vi "删除用户.vi"(6 "用户名-refnum-in":refnum<vi>, 8 "用户类别-refnum-in":refnum<vi>, 9 "管理人员1+密码":string[][](array[string]), 10 "操作人员0+密码":string[][](array[string]), 11 "密码文件路径":path=path "E:/LabVIEW Data/盾构/default") -> (2 "管理人员1+密码_out":string[][](array[string]), 3 "操作人员0+密码_out":string[][](array[string]))   [LabVIEW 2018]
panel:
  in  "用户名":u16(ring) caption="请在此选择用户名" items=["1", "2"]
  in  "用户类别":u8(ring) caption="请在此选择用户类别" items=["操作人员", "管理人员"]
  in  "请输入密码":string
  in  "返回":bool
  in  "删除":bool
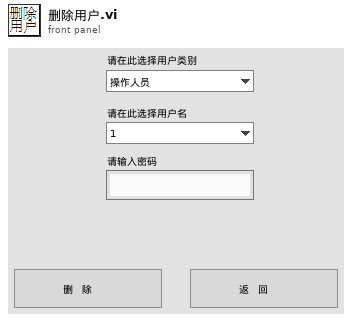
[diagram p1: front panel]
types:
  T1 = enum8{"Enabled", "Disabled", "Disabled and Grayed Out"}
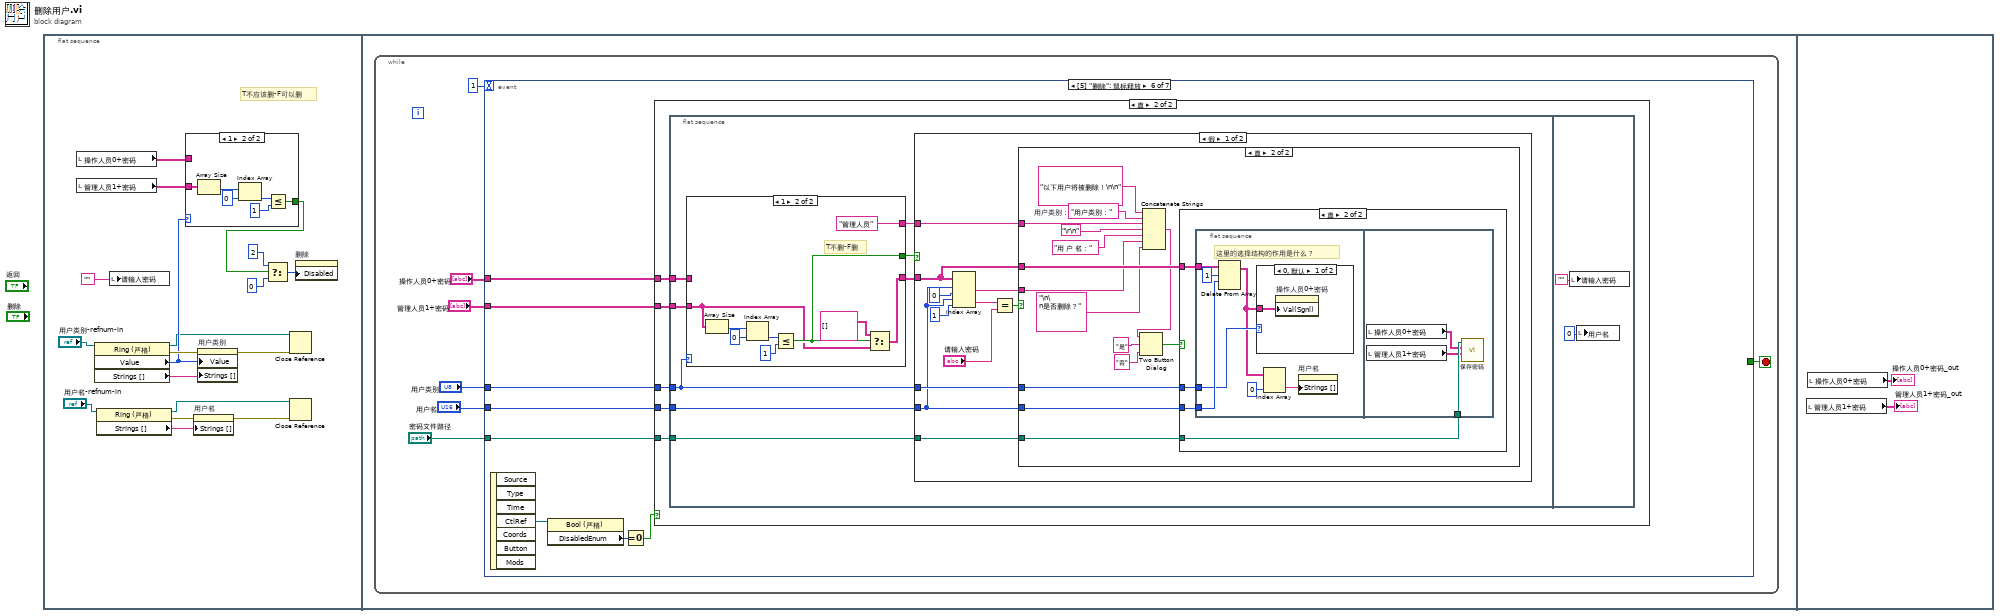
[diagram p0: block diagram]
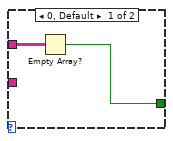
[diagram p2: hidden frame]
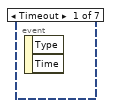
[diagram p3: hidden frame]
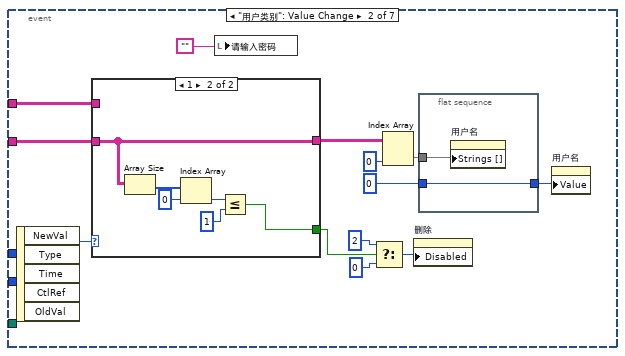
[diagram p4: hidden frame]
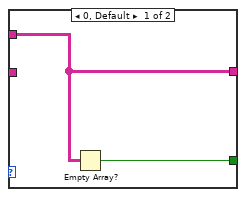
[diagram p5: hidden frame]
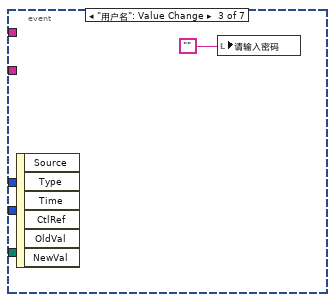
[diagram p6: hidden frame]
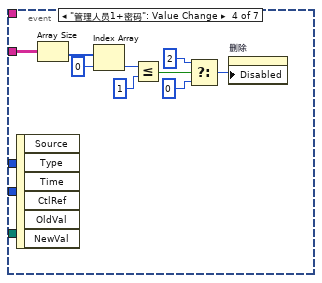
[diagram p7: hidden frame]
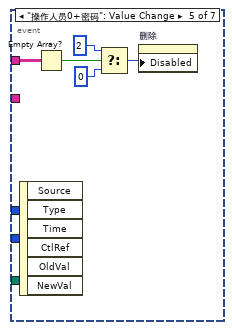
[diagram p8: hidden frame]
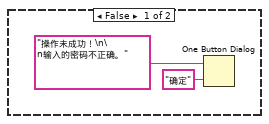
[diagram p10: hidden frame]
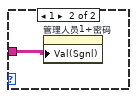
[diagram p12: hidden frame]
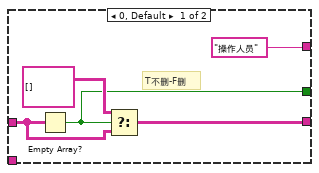
[diagram p14: hidden frame]
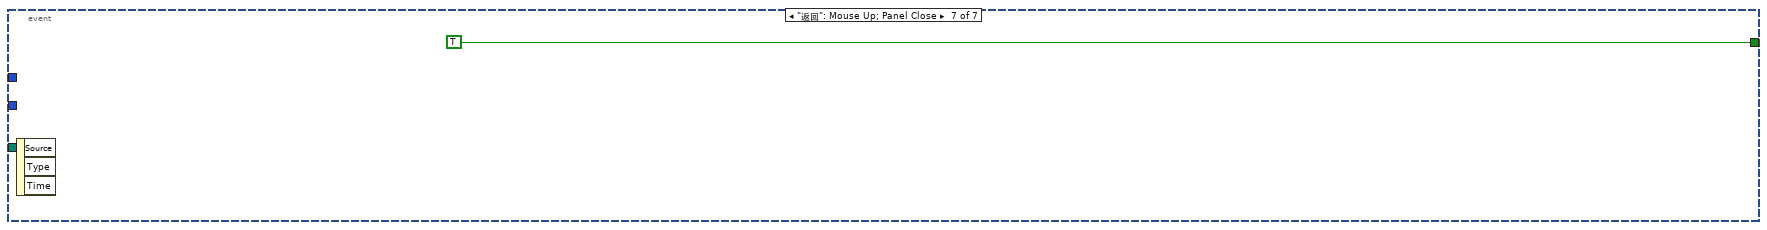
[diagram p15: hidden frame]
diagram:
  n1 = flat-sequence {
    frame #0 {
      # "T不应该删-F可以删"
      n2 = local read "操作人员0+密码"() -> (w10:string[][])
      n3 = local read "管理人员1+密码"() -> (w11:string[][])
      n4 = property class="Ring (严格)"(reference="用户类别-refnum-in") -> (reference out=w3:refnum<vi>, error out=w13:errorcluster, "Value"=w12:u8, "Strings []"=w17:string[])  [unwired: 1 in]
      n5 = property class="Ring (严格)"(reference="用户名-refnum-in") -> (reference out=w1:refnum<vi>, error out=w15:errorcluster, "Strings []"=w14:string[])  [unwired: 1 in]
      n6 = local write "请输入密码"("") -> ()
      n7 = case shown="1" w12 {
        tunnel: w10 -> [w20 _]
        tunnel: w11 -> [_ w21]
        tunnel: [w19 w22] -> w6
        frame 0, Default {
          n8 = Empty Array?(array=w20) -> (empty?=w19:bool)
        }
        frame 1 {
          n9 = Array Size(array=w21) -> (size(s)=w26:i32[])
          n10 = Index Array(array=w26, index=0 ("索引")) -> (element=w24:i32)
          n11 = Less Or Equal?(x=w24, y=1) -> (x <= y?=w22:bool)
        }
      }
      n12 = property on="用户名" class="Ring (严格)"(error in=w15, "Strings []"=w14) -> (error out=w2:errorcluster)  [unwired: 1 in, 1 out]
      n13 = property on="用户类别" class="Ring (严格)"(error in=w13, "Value"=w12, "Strings []"=w17) -> (error out=w4:errorcluster)  [unwired: 1 in, 1 out]
      n14 = Select(t=u8 2 ("禁用"), s=w6, f=u8 0 ("禁用")) -> (s? t:f=w7:u8)
      n15 = Close Reference(reference=w3, error in (no error)=w4) -> ()  [unwired: 1 out]
      n16 = Close Reference(reference=w1, error in (no error)=w2) -> ()  [unwired: 1 out]
      n17 = property on="删除" class="Bool (严格)"("Disabled"=w7) -> ()  [unwired: 2 in, 2 out]
    }
    frame #1 {
      n18 = while {
        stop <- w32 stop-if-true
        n19 = event shown="[5] \"删除\": 鼠标释放" {
          selector: _ -> [_ _ _ _ _ _ _]
          dyn-events: _ -> [_ _ _ _ _ _ _]
          timeout: 1 -> [_ _ _ _ _ _ _]
          tunnel: "操作人员0+密码" -> [_ w39 _ _ w71 w79 _]
          tunnel: "管理人员1+密码" -> [_ w38 _ w62 _ w78 _]
          tunnel: "用户类别" -> [_ _ _ _ _ w76 _]
          tunnel: "密码文件路径" -> [_ _ _ _ _ w75 _]
          tunnel: [_ _ _ _ _ _ TRUE] -> w32
          tunnel: "用户名" -> [_ _ _ _ _ w77 _]
          event Timeout {
            n20 = event-data() -> ()  [unwired: 1 in, 2 out]
          }
          event "用户类别": Value Change {
            n21 = event-data() -> ("NewVal"=w46:u8)  [unwired: 1 in, 4 out]
            n22 = case shown="1" w46 {
              tunnel: w39 -> [w50 _]
              tunnel: [w50 w52] -> w40
              tunnel: w38 -> [_ w52]
              tunnel: [w49 w51] -> w34
              frame 0, Default {
                n23 = Empty Array?(array=w50) -> (empty?=w49:bool)
              }
              frame 1 {
                n24 = Array Size(array=w52) -> (size(s)=w53:i32[])
                n25 = Index Array(array=w53, index=0 ("索引")) -> (element=w55:i32)
                n26 = Less Or Equal?(x=w55, y=1) -> (x <= y?=w51:bool)
              }
            }
            n27 = local write "请输入密码"("") -> ()
            n28 = Select(t=u8 2 ("禁用"), s=w34, f=u8 0 ("禁用")) -> (s? t:f=w35:u8)
            n29 = Index Array(array=w40, index (col)=0 ("禁用的索引 (col)")) -> (element=w45:string[])  [unwired: 1 in]
            n30 = property on="删除" class="Bool (严格)"("Disabled"=w35) -> ()  [unwired: 2 in, 2 out]
            n31 = flat-sequence {
              tunnel: w45 -> [w48]
              tunnel: [w47] -> w42
              tunnel: u16 0 ("禁用的索引 (col)") -> [w47]
              frame #0 {
                n32 = property on="用户名" class="Ring (严格)"("Strings []"=w48) -> ()  [unwired: 2 in, 2 out]
              }
            }
            n33 = property on="用户名" class="Ring (严格)"("Value"=w42) -> ()  [unwired: 2 in, 2 out]
          }
          event "用户名": Value Change {
            n34 = event-data() -> ()  [unwired: 1 in, 6 out]
            n35 = local write "请输入密码"("") -> ()
          }
          event "管理人员1+密码": Value Change {
            n36 = event-data() -> ()  [unwired: 1 in, 6 out]
            n37 = Array Size(array=w62) -> (size(s)=w63:i32[])
            n38 = Index Array(array=w63, index=0 ("索引")) -> (element=w65:i32)
            n39 = Less Or Equal?(x=w65, y=1) -> (x <= y?=w58:bool)
            n40 = Select(t=u8 2 ("禁用"), s=w58, f=u8 0 ("禁用")) -> (s? t:f=w61:u8)
            n41 = property on="删除" class="Bool (严格)"("Disabled"=w61) -> ()  [unwired: 2 in, 2 out]
          }
          event "操作人员0+密码": Value Change {
            n42 = event-data() -> ()  [unwired: 1 in, 6 out]
            n43 = Empty Array?(array=w71) -> (empty?=w67:bool)
            n44 = Select(t=u8 2 ("禁用"), s=w67, f=u8 0 ("禁用")) -> (s? t:f=w70:u8)
            n45 = property on="删除" class="Bool (严格)"("Disabled"=w70) -> ()  [unwired: 2 in, 2 out]
          }
          event "删除": Mouse Up {
            n46 = event-data() -> ("CtlRef"=w74:refnum<vi>)  [unwired: 1 in, 6 out]
            n47 = property class="Bool (严格)"(reference=w74) -> ("DisabledEnum"=w73:T1)  [unwired: 1 in, 2 out]
            n48 = Equal To 0?(x=w73) -> (x = 0?=w72:bool)
            n49 = case shown="真" w72 {
              tunnel: w79 -> [_ w84]
              tunnel: w78 -> [_ w83]
              tunnel: w77 -> [_ w82]
              tunnel: w76 -> [_ w81]
              tunnel: w75 -> [_ w80]
              frame False {
              }
              frame True {
                n50 = flat-sequence {
                  tunnel: w84 -> [w92]
                  tunnel: w83 -> [w91]
                  tunnel: w82 -> [w88]
                  tunnel: w81 -> [w87]
                  tunnel: w80 -> [w86]
                  frame #0 {
                    n51 = case shown="1" w87 {
                      tunnel: w92 -> [w141 _]
                      tunnel: [w139 w143] -> w89
                      tunnel: w91 -> [_ w144]
                      tunnel: [w138 w145] -> w90
                      tunnel: ["操作人员" "管理人员"] -> w85
                      frame 0, Default {
                        # "T不删-F删"
                        n52 = Empty Array?(array=w141) -> (empty?=w138:bool)
                        n53 = Select(t=string[][] [] ("操作人员0+密码 2"), s=w138, f=w141) -> (s? t:f=w139:string[][])
                      }
                      frame 1 {
                        # "T不删-F删"
                        n54 = Array Size(array=w144) -> (size(s)=w150:i32[])
                        n55 = Index Array(array=w150, index=0 ("索引")) -> (element=w148:i32)
                        n56 = Less Or Equal?(x=w148, y=1) -> (x <= y?=w145:bool)
                        n57 = Select(t=string[][] [] ("操作人员0+密码 2"), s=w145, f=w144) -> (s? t:f=w143:string[][])
                      }
                    }
                    n58 = case shown="假" w90 {
                      tunnel: w89 -> [w100 _]
                      tunnel: w88 -> [w96 _]
                      tunnel: w87 -> [w99 _]
                      tunnel: w86 -> [w98 _]
                      tunnel: w85 -> [w97 _]
                      frame False {
                        n59 = Index Array(array=w100, index (row) #1=w96, index (col) #1=0 ("禁用的索引 (col)"), index (row) #2=w96, index (col) #2=1 ("禁用的索引 (col)")) -> (element #1=w93:string, element #2=w94:string)
                        n60 = Equal?(x=w94, y="请输入密码") -> (x = y?=w101:bool)
                        n61 = case shown="真" w101 {
                          tunnel: w100 -> [_ w120]
                          tunnel: w96 -> [_ w119]
                          tunnel: w99 -> [_ w118]
                          tunnel: w98 -> [_ w117]
                          tunnel: w97 -> [_ w109]
                          tunnel: w93 -> [_ w108]
                          frame False {
                            n62 = One Button Dialog(message="操作未成功！\n\n输入的密码不正确。" ("消息"), button name ("OK")="确定" ("按钮名称（“确定”）")) -> ()  [unwired: 1 out]
                          }
                          frame True {
                            w113 = "用户类别："  # 用户类别：
                            n63 = Concatenate Strings("以下用户将被删除！\n\n", w113, w109, "\r\n", "用 户 名：", w108, "\n\n是否删除？") -> (w106:string)
                            n64 = Two Button Dialog(message=w106, 1:"否" ("按钮名称（“确定”）"), 2:"是" ("按钮名称（“确定”）")) -> (T button?=w116:bool)
                            n65 = case shown="真" w116 {
                              tunnel: w120 -> [_ w124]
                              tunnel: w119 -> [_ w123]
                              tunnel: w118 -> [_ w122]
                              tunnel: w117 -> [_ w121]
                              frame False {
                              }
                              frame True {
                                n66 = flat-sequence {
                                tunnel: w124 -> [w131]
                                tunnel: w123 -> [w129]
                                tunnel: w122 -> [w128]
                                tunnel: w121 -> [w136]
                                frame #0 {
                                # "这里的选择结构的作用是什么？"
                                n67 = Delete From Array(array=w131, length=1 ("长度"), index (row)=w129) -> (array with subset deleted=w127:string[][])  [unwired: 1 in, 1 out]
                                n68 = case shown="0, 默认" w128 {
                                tunnel: w127 -> [w132 w133]
                                frame 0, Default {
                                n69 = property on="操作人员0+密码" class="Arr (严格)"("Val(Sgnl)"=w132) -> ()  [unwired: 2 in, 2 out]
                                }
                                frame 1 {
                                n70 = property on="管理人员1+密码" class="Arr (严格)"("Val(Sgnl)"=w133) -> ()  [unwired: 2 in, 2 out]
                                }
                                }
                                n71 = Index Array(array=w127, index (col)=0 ("禁用的索引 (col)")) -> (element=w125:string[])  [unwired: 1 in]
                                n72 = property on="用户名" class="Ring (严格)"("Strings []"=w125) -> ()  [unwired: 2 in, 2 out]
                                }
                                frame #1 {
                                n73 = local read "操作人员0+密码"() -> (w135:string[][])
                                n74 = local read "管理人员1+密码"() -> (w134:string[][])
                                n75 = call "保存密码.vi"("密码文件路径"=w136, "操作人员0+密码"=w135, "管理人员1+密码"=w134) -> ()  [unwired: 4 in, 1 out]
                                }
                                }
                              }
                            }
                          }
                        }
                      }
                      frame True {
                      }
                    }
                  }
                  frame #1 {
                    n76 = local write "请输入密码"("") -> ()
                    n77 = local write "用户名"(u16 0) -> ()
                  }
                }
              }
            }
          }
          event "返回": Mouse Up; Panel Close {
            n78 = event-data() -> ()  [unwired: 1 in, 3 out]
          }
        }
      }
    }
    frame #2 {
      n79 = local read "管理人员1+密码"() -> (→"管理人员1+密码_out":string[][])
      n80 = local read "操作人员0+密码"() -> (→"操作人员0+密码_out":string[][])
    }
  }
